vi "ScriptWrite.vi"(0 "Marker shape":string, 1 "Marker size":i32, 2 "Open PDF":bool=TRUE, 3 "Open in MATLAB":bool=TRUE, 4 "Traces colors string (RGB)":string[](array[string]), 5 "PDF file path":path, 7 "Script.m path":path, 8 "Traces.txt":string, 9 "PNG file name":string, 11 "Colors error":errorcluster) -> (17 "ScriptWrite error":errorcluster, 21 "Script.m":string)   [LabVIEW 2023]
panel:
  out "resulting string 2":string
  out "s? t:f":string
  out "concatenated string":string
  in  "User interface":T1(tab)
  in  "User entries":enum32{""}(tab)
  in  "Customization":enum32{"Customization"}(tab)
  in  "Colors":enum32{"Colors"}(tab)
  in  "Size":enum32{"Size"}(tab)
  out "resulting string 1":string
  in  "Loop FOR 1":enum32{"Loop FOR 1"}(tab)
  in  "Arrays":enum32{"Arrays"}(tab)
  in  "Script.m":enum32{"Script.m"}(tab)
  out "Colors string":string
  in  "Extract.c output string scan":enum32{"Extract.c output string scan"}(tab)
  in  "T: tt1 tt2 tt3 ...":enum32{"T: tt1 tt2 tt3 ..."}(tab)
  in  "C: cc":enum32{"C: cc"}(tab)
  in  "Loop FOR 2":enum32{"Loop FOR 2"}(tab)
  in  "LabVIEW":enum32{"LabVIEW"}(tab)
  in  "MATLAB":enum32{"MATLAB"}(tab)
  in  "C":enum32{"C"}(tab)
  in  "MATLAB":enum32{"MATLAB"}(tab)
  in  "C":enum32{"C"}(tab)
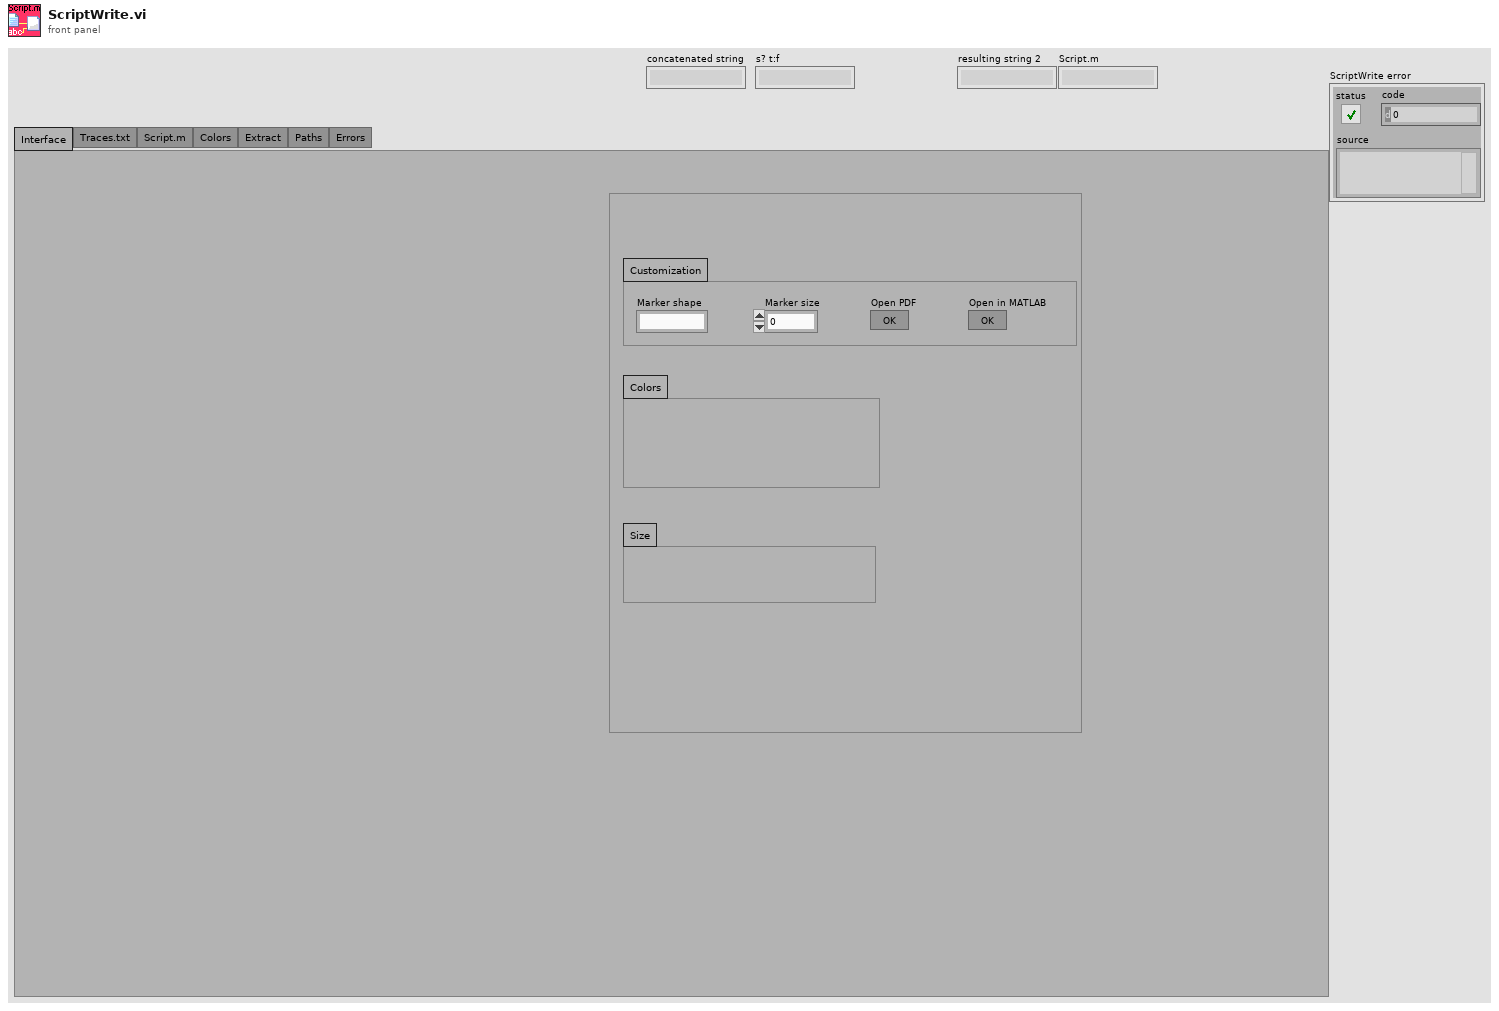
[diagram p1: front panel]
types:
  T1 = enum32{"Interface", "Traces.txt", "Script.m", "Colors", "Extract", "Paths", "Errors"}
  T2 = enum16{"open", "replace", "create", "open or create", "replace or create", "replace or create with confirmation"}
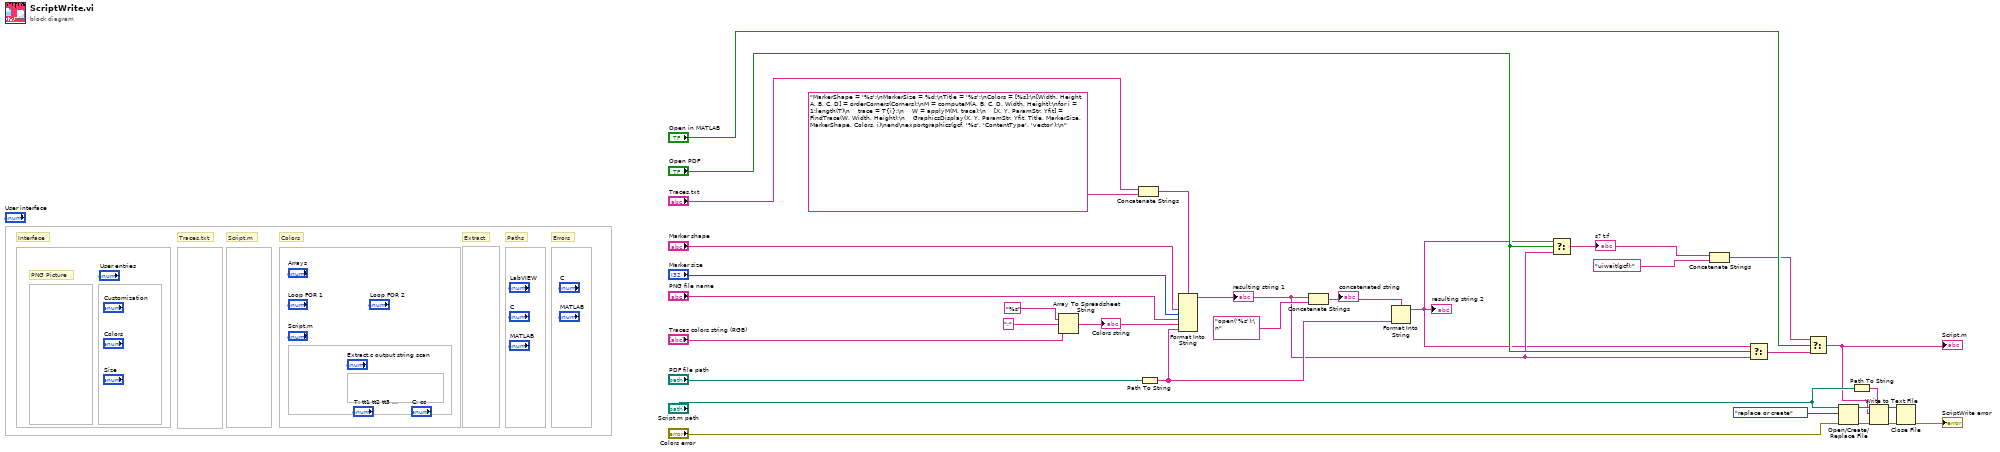
[diagram p0: block diagram]
diagram:
  # "PNG Picture"
  # "Errors"
  # "Paths"
  # "Extract"
  # "Colors"
  # "Script.m"
  # "Traces.txt"
  # "Interface"
  n1 = Array To Spreadsheet String(delimiter (Tab)=";", array="Traces colors string (RGB)", 3:"%s" ("format string")) -> (spreadsheet string=w19:string)
  "Colors string" <- w19
  n2 = Concatenate Strings("Traces.txt", "MarkerShape = '%s';\nMarkerSize = %d;\nTitle = '%s';\nColors = [%s];\n[Width, Height, A, B, C, D] = orderCorners(Corners);\nM = computeM(A, B, C, D, Width, Height);\nfor i = 1:length(T)\n    trace = T{i};\n    W = applyM(M, trace);\n    [X, Y, ParamStr, Yfit] = FindTrace(W, Width, Height);\n    GraphicsDisplay(X, Y, ParamStr, Yfit, Title, MarkerSize, MarkerShape, Colors, i)\nend\nexportgraphics(gcf, '%s', 'ContentType', 'vector');\n" ("initial string")) -> (w13:string)
  n3 = Path To String(path="PDF file path") -> (string=w8:string)
  n4 = Format Into String(format string=w13, "Marker shape", "Marker size", "PNG file name", w19, w8) -> (resulting string=w5:string)  [unwired: 2 in, 1 out]
  "resulting string 1" <- w5
  n5 = Concatenate Strings(w5, "open('%s');\n" ("initial string")) -> (w10:string)
  "concatenated string" <- w10
  n6 = Format Into String(format string=w10, w8) -> (resulting string=w4:string)  [unwired: 2 in, 1 out]
  "resulting string 2" <- w4
  n7 = Select(t=w4, s="Open PDF", f=w5) -> (s? t:f=w3:string)
  "s? t:f" <- w3
  n8 = Concatenate Strings(w3, "uiwait(gcf);" ("initial string")) -> (w1:string)
  n9 = Select(t=w4, s="Open PDF", f=w5) -> (s? t:f=w7:string)
  n10 = Select(t=w1, s="Open in MATLAB", f=w7) -> (s? t:f=w9:string)
  "Script.m" <- w9
  n11 = Open/Create/Replace File(file path (use dialog)="Script.m path", error in="Colors error", operation (0:open)=T2."replace or create") -> (refnum out=w32:refnum<file>, error out=w30:errorcluster)  [unwired: 3 in, 1 out]
  n12 = Path To String(path="Script.m path") -> (string=w27:string)
  n13 = Write to Text File(prompt (Choose or enter file path)=w27, file (use dialog)=w32, text=w9, error in=w30) -> (refnum out=w28:refnum<file>, error out=w29:errorcluster)  [unwired: 1 out]
  n14 = Close File(refnum=w28, error in=w29) -> (error out=→"ScriptWrite error":errorcluster)  [unwired: 1 out]
